vi "stimulus_intensity_to_red_blue_color_together.vi"(1 "StimulusIntensityForFrame":sgl[](array[numeric])) -> (0 "StimulusColorForFrame":sgl)   [LabVIEW 2019]
uses:
  ParametersGlobal.vi
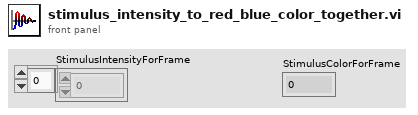
[diagram p1: front panel]
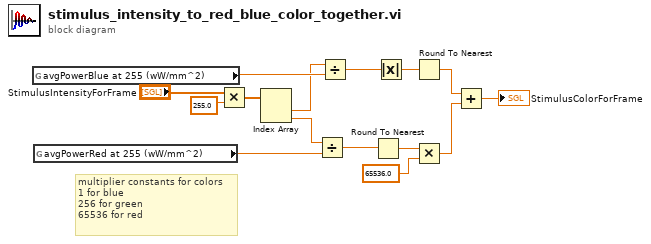
[diagram p0: block diagram]
diagram:
  # "multiplier constants for colors\n1 for blue\n256 for green\n65536 for red"
  n1 = global read "ParametersGlobal.vi" "avgPowerBlue at 255 (wW/mm^2)"() -> (w13:sgl)
  n2 = global read "ParametersGlobal.vi" "avgPowerRed at 255 (wW/mm^2)"() -> (w12:sgl)
  n3 = Multiply(x="StimulusIntensityForFrame", y=sgl 255.0) -> (x*y=w4:sgl[])
  n4 = Index Array(array=w4) -> (element #1=w3:sgl, element #2=w2:sgl)  [unwired: 2 in]
  n5 = Divide(x=w2, y=w12) -> (x/y=w7:sgl)
  n6 = Divide(x=w3, y=w13) -> (x/y=w6:sgl)
  n7 = Round To Nearest(number=w7) -> (nearest integer value=w11:sgl)
  n8 = Absolute Value(x=w6) -> (abs(x)=w9:sgl)
  n9 = Round To Nearest(number=w9) -> (nearest integer value=w8:sgl)
  n10 = Multiply(x=w11, y=sgl 65536.0) -> (x*y=w10:sgl)
  n11 = Add(x=w8, y=w10) -> (x+y=→"StimulusColorForFrame":sgl)
